vi "CC Get All Files for Image.vi"(8 "error in (no error)":errorcluster, 11 "path":path) -> (0 "error out":errorcluster, 3 "Files for image":path[](array[path]))   [LabVIEW 2024]
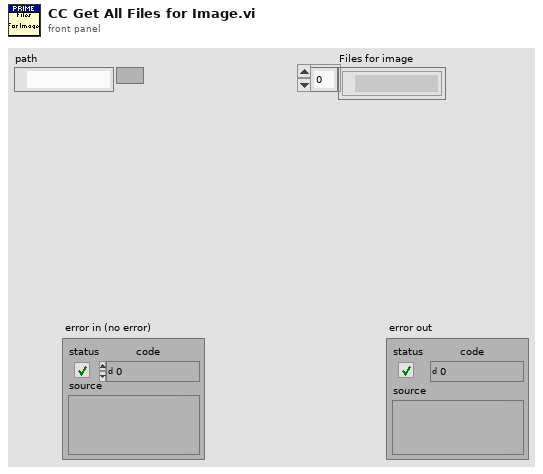
[diagram p1: front panel]
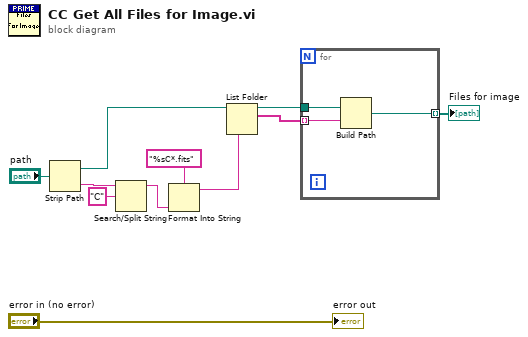
[diagram p0: block diagram]
diagram:
  n1 = Strip Path(path="path") -> (stripped path=w6:path, name=w10:string)
  n2 = Search/Split String(string=w10, search string/char (-)="C") -> (substring before match=w7:string)  [unwired: 1 in, 2 out]
  n3 = Format Into String(format string="%sC*.fits", w7) -> (resulting string=w5:string)  [unwired: 2 in, 1 out]
  n4 = List Folder(path=w6, pattern=w5) -> (path out=w3:path, filenames=w2:string[])  [unwired: 2 in, 2 out]
  n5 = for {
    tunnel: w3 -> [w14]
    tunnel: w2 -> [w13] mode=indexing
    tunnel: [w12] -> w1 mode=indexing
    n6 = Build Path(base path=w14, name or relative path=w13) -> (appended path=w12:path)
  }
  "Files for image" <- w1
  "error out" <- "error in (no error)"
